vi "Runtime Test.vi"() -> ()   [LabVIEW 2018, in "Benchmark PID tests.lvlib"]
doc: "This VI shows an example for how to test the Runtime functionality of the module. This will need to be modified according to module functionality."
uses:
  Benchmark PID tests.lvlib
  <vilib>/NI/Tag Bus Module Framework/channel/TBM channel.lvclass
  C:/Program Files (x86)/National Instruments/LabVIEW 2018/vi.lib/NI/Tag Bus/tag/tag descriptor.lvclass
  <vilib>/NI/Tag Bus Module Framework/channel/channel classification.ctl
  module/execution/Benchmark PID runtime.lvclass
  <vilib>/NI/Tag Bus/tag/tag descriptor.lvclass/tag descriptor.ctl
  <vilib>/NI/Tag Bus Module Framework/channel/TBM channel.lvclass/TBM channel.ctl
  <vilib>/NI/Tag Bus/dictionary/data dictionary.lvclass/data dictionary.ctl
  <vilib>/NI/Tag Bus/dictionary/lookup polymorphs/locate double.vi
  <vilib>/NI/Tag Bus/table/data polymorphs/write one/write Double.vi
  <vilib>/NI/Tag Bus/table/data polymorphs/read one/read Double.vi
  <vilib>/NI/Tag Bus/dictionary/search/find data index.vi
  <vilib>/NI/Tag Bus/dictionary/search/search string list.vi
  module/configuration/Benchmark PID configuration.lvclass
  C:/Program Files (x86)/National Instruments/LabVIEW 2018/vi.lib/NI/Tag Bus Module Framework/module configuration/TBM module configuration.lvclass
  <vilib>/NI/Tag Bus/dictionary/tag not found.vi
  <vilib>/NI/Tag Bus/dictionary/data dictionary.lvclass
  <vilib>/NI/Tag Bus/table/data table.lvlib
  <vilib>/NI/Tag Bus/tag/tag descriptor.lvclass
panel:
  out "Array 2":T1[](array[typedef])
  out "Array":string[](array[string])
  out "channels":refnum<class "TBM channel.lvclass">[](array[class])
  in  "Variable":dbl format="%#_13g"
  out "Output":dbl
  in  "Setpoint":dbl
  out "error":errorcluster
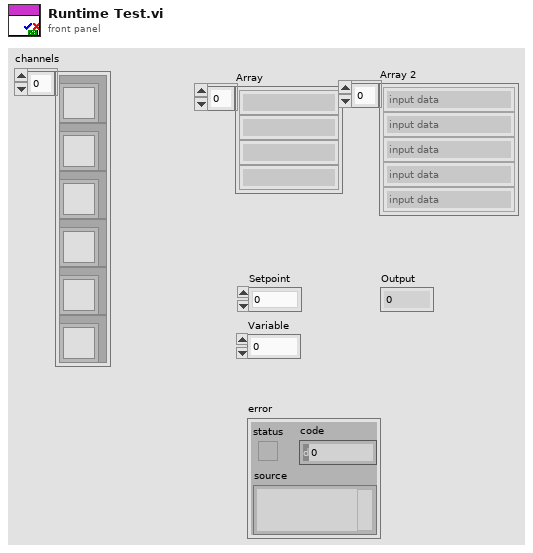
[diagram p1: front panel]
types:
  T1 = typedef "TBM channel.lvclass/channel classification.ctl" = enum16{"input data", "output data", "processing parameter", "processing result"}
  T2 = typedef "TBM channel.lvclass/data tables.ctl" = cluster{"input data":T3, "processing parameter":T3, "processing result":T3, "output data":T3}
  T3 = typedef "tag bus.lvlib/dictionary table pair.ctl" = cluster{"data dictionary":refnum<class "data dictionary.lvclass">, "data table":T4}
  T4 = typedef "tag bus.lvlib/data table.lvlib/data table.ctl" = cluster{"Double":dbl[], "Single":sgl[], "I64":i64[], "I32":i32[], "I16":i16[], "I8":i8[], "U64":u64[], "U32":u32[], "U16":u16[], "U8":u8[], "Boolean":bool[], "String":string[], "Array of Double":cluster{"DBL Array":dbl[]}[], "Array of Single":cluster{"SGL Array":sgl[]}[], "Array of I64":cluster{"I64 Array":i64[]}[], "Array of I32":cluster{"I32 Array":i32[]}[], "Array of I16":cluster{"I16 Array":i16[]}[], "Array of I8":cluster{"I8 Array":i8[]}[], "Array of U64":cluster{"U64 Array":u64[]}[], "Array of U32":cluster{"U32 Array":u32[]}[], "Array of U16":cluster{"U16 Array":u16[]}[], "Array of U8":cluster{"U8 Array":u8[]}[], "Array of Boolean":cluster{"Boolean Array":bool[]}[], "Array of String":cluster{"String Array":string[]}[]}
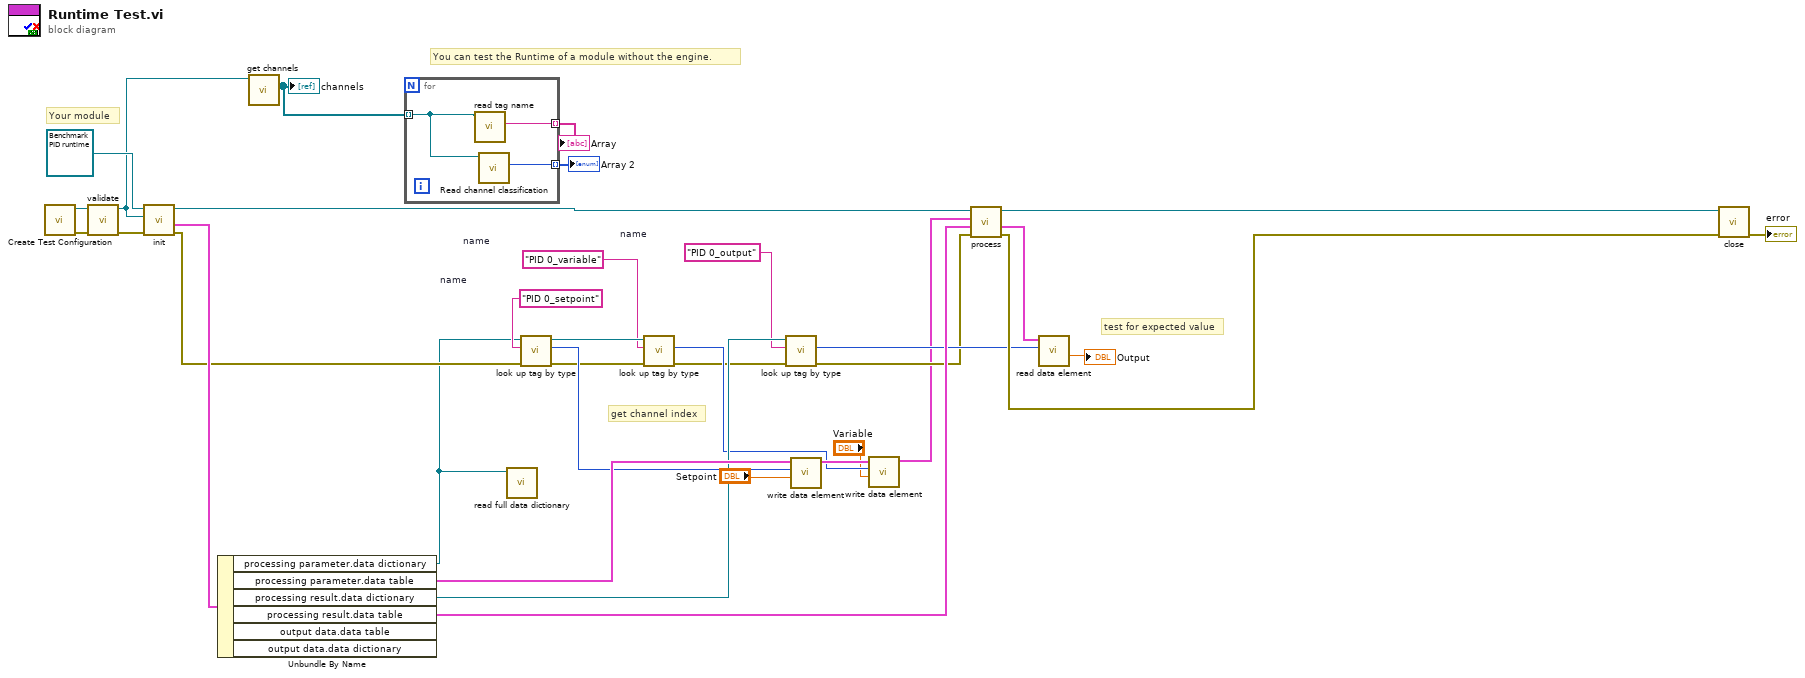
[diagram p0: block diagram]
diagram:
  w12 = "PID 0_variable"  # name
  w18 = "PID 0_setpoint"  # name
  w20 = "PID 0_output"  # name
  # "test for expected value"
  # "get channel index"
  # "You can test the Runtime of a module without the engine."
  # "Your module"
  n1 = call "Create Test Configuration.vi"() -> ("error out"=w31:errorcluster, "Module Configuration"=w32:refnum<class "Benchmark PID configuration.lvclass">)  [unwired: 6 in, 4 out]
  n2 = call-dynamic "validate.vi"("error in"=w31, "Benchmark PID configuration in"=w32) -> ("error out"=w33:errorcluster, "Benchmark PID configuration out"=w6:refnum<class "Benchmark PID configuration.lvclass">)  [unwired: 8 in]
  n3 = call-dynamic "init.vi"("error in"=w33, "TBM module configuration in"=w6, "Benchmark PID runtime in"=refnum<class "Benchmark PID runtime.lvclass"> refnum ("tag bus configurable plugin module")) -> ("error out"=w24:errorcluster, "data allocations"=w25:T2, "Benchmark PID runtime out"=w26:refnum<class "Benchmark PID runtime.lvclass">)  [unwired: 5 in, 1 out]
  n4 = Unbundle By Name(w25) -> ("processing parameter.data dictionary"=w7:refnum<class "data dictionary.lvclass">, "processing parameter.data table"=w30:T4, "processing result.data dictionary"=w28:refnum<class "data dictionary.lvclass">, "processing result.data table"=w27:T4)  [unwired: 2 out]
  n5 = call-dynamic "get channels.vi"("Benchmark PID configuration in"=w6) -> ("channels"=w3:refnum<class "TBM channel.lvclass">[])  [unwired: 9 in, 1 out]
  "channels" <- w3
  n6 = for {
    tunnel: w3 -> [w37] mode=indexing
    tunnel: [w36] -> w2 mode=indexing
    tunnel: [w35] -> w1 mode=indexing
    n7 = call <vilib>:"read tag name.vi"("system tag in"=w37) -> ("name"=w36:string)  [unwired: 8 in, 2 out]
    n8 = call <vilib>:"Read channel classification.vi"("channel in"=w37) -> ("channel classification"=w35:T1)  [unwired: 8 in, 2 out]
  }
  "Array" <- w2
  "Array 2" <- w1
  n9 = call <vilib>:"read full data dictionary.vi"("data dictionary in"=w7) -> ()  [unwired: 8 in, 3 out]
  n10 = call-poly <vilib>:"look up tag by type.vi"("error in"=w24, "name"=w18, "data dictionary in"=w7) -> ("error out"=w5:errorcluster, "index"=w19:i32, "data dictionary out"=w13:refnum<class "data dictionary.lvclass">)  [unwired: 6 in]
  n11 = call-poly <vilib>:"look up tag by type.vi"("error in"=w5, "name"=w12, "data dictionary in"=w13) -> ("error out"=w4:errorcluster, "index"=w9:i32)  [unwired: 6 in, 1 out]
  n12 = call-poly <vilib>:"look up tag by type.vi"("error in"=w4, "name"=w20, "data dictionary in"=w28) -> ("error out"=w16:errorcluster, "index"=w21:i32)  [unwired: 6 in, 1 out]
  n13 = call-poly <vilib>:"write data element.vi"("value"="Setpoint", "index"=w19, "data table in"=w30) -> ("data table out"=w11:T4)  [unwired: 8 in]
  n14 = call-poly <vilib>:"write data element.vi"("value"="Variable", "index"=w9, "data table in"=w11) -> ("data table out"=w10:T4)  [unwired: 8 in]
  n15 = call-dynamic "process.vi"("error in"=w16, "result allocation"=w27, "parameters"=w10, "module in"=w26) -> ("error out"=w22:errorcluster, "results"=w17:T4, "module out"=w23:refnum<class "Benchmark PID runtime.lvclass">)  [unwired: 4 in, 1 out]
  n16 = call-poly <vilib>:"read data element.vi"("index"=w21, "data table in"=w17) -> ("value"=→"Output":dbl)  [unwired: 8 in, 1 out]
  n17 = call-dynamic "close.vi"("error in"=w22, "Benchmark PID runtime in"=w23) -> ("error out"=→"error":errorcluster)  [unwired: 9 in]
